vi "PopulateTree.vi"(8 "error in (no error)":errorcluster, 10 "Array":T1(array[cluster]), 11 "TreeControl in":refnum<vi>) -> (0 "error out":errorcluster)   [LabVIEW 2018]
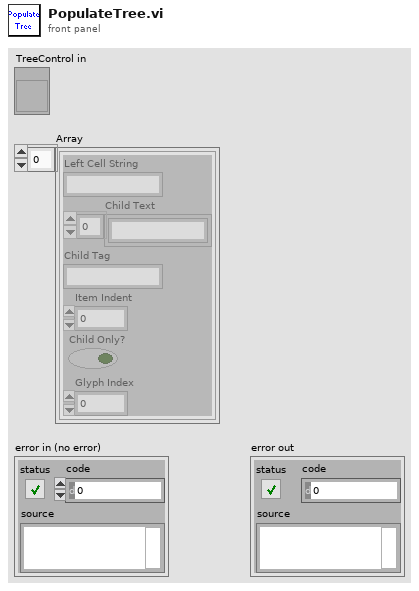
[diagram p1: front panel]
types:
  T1 = cluster{"Left Cell String":string, "Child Text":string[], "Child Tag":string, "Item Indent":i32, "Child Only?":bool, "Glyph Index":i32}[]
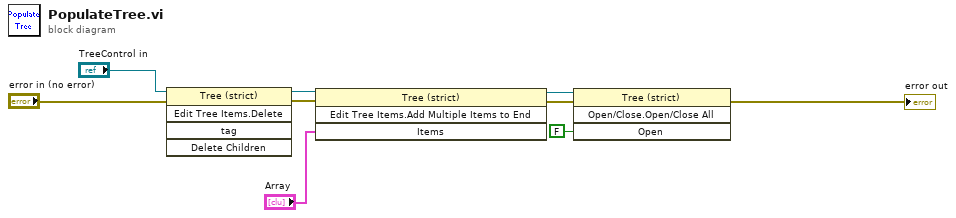
[diagram p0: block diagram]
diagram:
  n1 = invoke on="Invoke Node" class="Tree (strict)" method="Edit Tree Items.Delete"(reference="TreeControl in", error in="error in (no error)") -> (reference out=w5:refnum<vi>, error out=w4:errorcluster)  [unwired: 3 in, 3 out]
  n2 = invoke on="Invoke Node" class="Tree (strict)" method="Edit Tree Items.Add Multiple Items to End"(reference=w5, error in=w4, "Items"="Array") -> (reference out=w6:refnum<vi>, error out=w7:errorcluster)  [unwired: 1 in, 2 out]
  n3 = invoke on="Invoke Node" class="Tree (strict)" method="Open/Close.Open/Close All"(reference=w6, error in=w7, "Open"=FALSE ("Open?")) -> (error out=→"error out":errorcluster)  [unwired: 1 in, 3 out]
